vi "2_PTLF_Classification_Model_Converter.vi"() -> ()   [LabVIEW 2020]
uses:
  <vilib>/Ngene/DeepLTK FPGA Addon/Toolkit/NNF_Host/Low_Level/Network_Converter/Controls/Range_Calculation_Specs.ctl
  <vilib>/Ngene/Deep Learning Toolkit/Toolkit/NN_Network/Controls/NN_Device.ctl
  <vilib>/Ngene/Deep Learning Toolkit/Toolkit/Deep_Learning_Toolkit_by_Ngene.lvlib
  <vilib>/Ngene/DeepLTK FPGA Addon/Toolkit/DeepLTK_FPGA_Addon.lvlib
panel:
  in  "Dataset Path":path=path "D:/Ngene/GitHub/deepltk_fpga_examples/3_PTLF_Classification(PXI,sbRIO)/Dataset/Test"
  out "error out":errorcluster
  in  "Wights file":path=path "D:/Ngene/GitHub/deepltk_fpga_examples/3_PTLF_Classification(PXI,sbRIO)/Models/0_PTLF_Classification_Original/PTLF_Classifier_weights_24_11_21__13_37_15.bin"
  in  "Configuration file":path=path "D:/Ngene/GitHub/deepltk_fpga_examples/3_PTLF_Classification(PXI,sbRIO)/Models/0_PTLF_Classification_Original/PTLF_Classifier_net_cfg_24_11_21__13_37_15.cfg"
  out "Generated_Files":path[](array[path])
  in  "Dest":path=path "D:/Ngene/GitHub/deepltk_fpga_examples/3_PTLF_Classification(PXI,sbRIO)/Models/1_PTLF_Classification_Converted"
  # "Overview: This example demonstrates the preparation process of pretrained PTLF model to be deployed on FPGA.\nIt consists of the following stages:\n1. Network optimization by merging applicable layers together.\n2. Per layer weights and output statistics calculation for optimal quantization on FPGA.\n3. Saving converted model together with statistical information to be used during the deployment.\nRequirements:\n•DeepLTK - Deep Learning Toolkit for LabVIEW (https://www.ngene.co/deep-learning-toolkit-for-labview)\n•DeepLTK FPGA Addon(https://www.ngene.co/deepltk-accelerator-for-fpga)\n•Sample dataset for reliable output statistic calculation. \nInstructions: \n1.\tProvide the path to the configuration file of a pretrained model in the \"Configuration File\" control.\n2.\tProvide the path to the weights file of a pretrained model in the \"Weights File\" control. \n3.\tProvide the path to the MNIST dataset used during training in the \"Dataset Path\" control. \n4.\tProvide the destination directory where the results will be stored in the \"Dest\" control.\n5.\tRun the VI and wait until all processes are completed.\n\nThe resulting files (Scalers .cfg, Weights .bin, and Configuration .cfg) will be stored at paths displayed in \"Generated_Files\" indicator.\nThis files will be used during inference process.\nMore Examples: https://github.com/ngenehub/deepltk_fpga_examples"
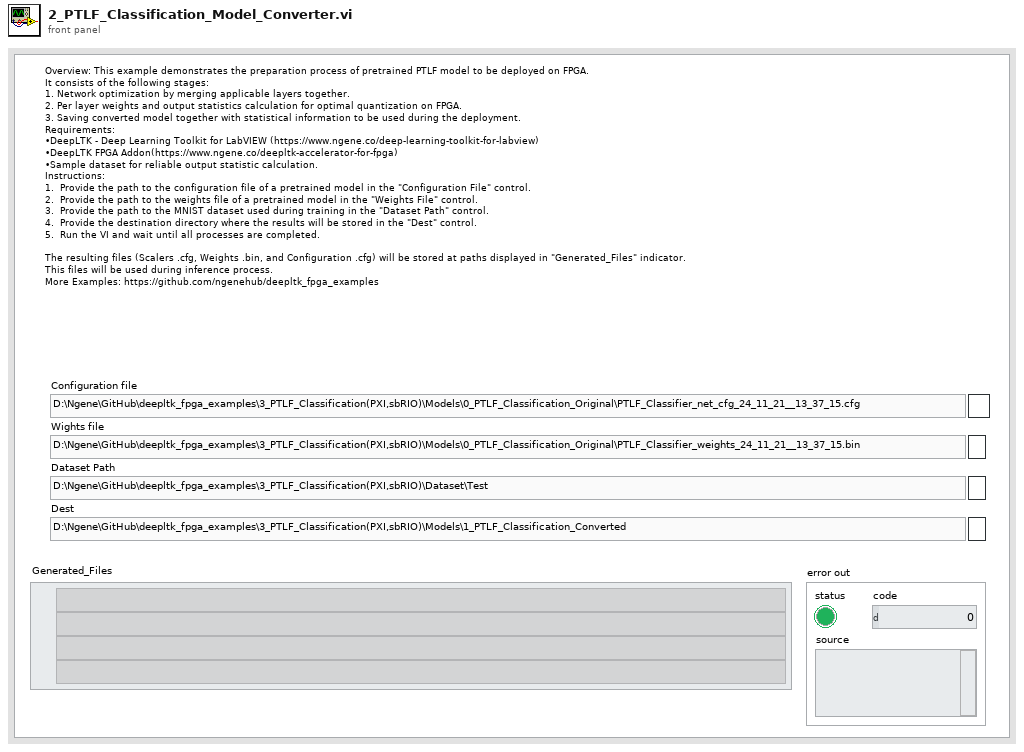
[diagram p1: front panel]
types:
  T1 = typedef "DeepLTK_FPGA_Addon.lvlib/Range_Calculation_Specs.ctl" = cluster{"# of Histogram Bins":i32, "Outputs Range Percentile(0.9999)":dbl, "Weights Range Percentile(0.9999)":dbl}
  T2 = typedef "Deep_Learning_Toolkit_by_Ngene.lvlib/NN_Device.ctl" = enum16{"CPU", "GPU"}
  T3 = typedef "Deep_Learning_Toolkit_by_Ngene.lvlib/NN_DataSets_All(In1D_Out1D).ctl" = cluster{"Train":T4, "Validation":T4, "Test":T4}
  T4 = typedef "Deep_Learning_Toolkit_by_Ngene.lvlib/NN_DataSet(In1D_Out1D).ctl" = cluster{"Inputs Ref.":variant, "Outputs Ref.":T5, "Dims_In":i32, "Dataset_Size":i32, "Dims_Out":i32, "Labels":string[], "File Paths":path[]}
  T5 = typedef "Deep_Learning_Toolkit_by_Ngene.lvlib/NN_Data_ref(2D_SGL).ctl" = refnum<data-value>
  T6 = typedef "Deep_Learning_Toolkit_by_Ngene.lvlib/NN_Config_Params.ctl" = cluster{"Name":string, "mBatch":i32, "NN_Train_Params":T7, "LR_Decay_Policy":T10, "Labels":string[], "Loss":T12}
  T7 = typedef "Deep_Learning_Toolkit_by_Ngene.lvlib/NN_Train_Params.ctl" = cluster{"Optimizer":T8, "Beta_1":sgl, "Beta_2":sgl, "Weight Decay(L1)":sgl, "Weight Decay(L2)":sgl, "Data_Sampling":T9}
  T8 = typedef "Deep_Learning_Toolkit_by_Ngene.lvlib/NN_Train_Optimizer.ctl" = enum16{"SGD", "Adam", "Adagrad", "Adadelta", "RMSProp", "Nesterov"}
  T9 = typedef "Deep_Learning_Toolkit_by_Ngene.lvlib/NN_Train_Data_Sampling.ctl" = enum16{"Random", "Sequential"}
  T10 = typedef "Deep_Learning_Toolkit_by_Ngene.lvlib/NN_LR_Policy_Cfg.ctl" = cluster{"Policy_Type":T11, "LR0":dbl, "k":sgl, "WarmUp_Policy":enum16{"Step", "Ramp"}, "WarmUp_Iter":i32, "WarmUp_Ratio":sgl}
  T11 = typedef "Deep_Learning_Toolkit_by_Ngene.lvlib/NN_LR_Policy_Type.ctl" = enum16{"Manual", "Step", "Exp", "1/t"}
  T12 = typedef "Deep_Learning_Toolkit_by_Ngene.lvlib/NN_Loss_Config_Params.ctl" = cluster{"Loss_Type":T13, "Loss_Conf_Params":variant}
  T13 = typedef "Deep_Learning_Toolkit_by_Ngene.lvlib/NN_Loss_Type.ctl" = enum16{"None", "MSE", "CrossEntropy", "YOLO_v2", "YOLO_v4"}
  T14 = typedef "Deep_Learning_Toolkit_by_Ngene.lvlib/NN_Layer_Config_Params.ctl" = cluster{"Layer_Type":T15, "Layer_Conf_Params":variant, "Input Layers":string[]}
  T15 = typedef "Deep_Learning_Toolkit_by_Ngene.lvlib/NN_Layer_Type.ctl" = enum16{"Input1D", "Input3D", "Conv1D", "Conv2D", "Conv2D_Adv", "MaxPool", "AvgPool", "UpSample", "DropOut3D", "ShortCut", "Concat", "SoftMax3D", "FC", "DropOut", "Softmax", "Flatten", "YOLO_v2", "YOLO_v4", "Activation", "BatchNormalization", "Unsupported"}
  T16 = typedef "Deep_Learning_Toolkit_by_Ngene.lvlib/NN.ctl" = cluster{"Name":string, "No of Layers":i32, "mBatch":i32, "Layers":T17[], "Dimty":T18, "Dims_In":T19, "Dims_Out":T19, "Working_Dir":path, "Train?":bool, "Train_Params":T7, "LR_Update_Policy":T10, "Session Data":T20, "Ground_truth":T21, "NNg_hdls":T22, "NN_Device":T2, "GPU Id":i32, "Labels":string[], "Receptive Field":T23[], "Loss_Type":T13, "Loss_Cfg_Prms":variant, "NNG_WS":T24}
  T17 = typedef "Deep_Learning_Toolkit_by_Ngene.lvlib/NN_Layer_ref.ctl" = refnum<data-value>
  T18 = typedef "Deep_Learning_Toolkit_by_Ngene.lvlib/NN_In_Out_Dim-ty.ctl" = enum8{"In1D_Out1D", "In3D_Out1D", "In3D_Out3D", "In3D_OutBBox"}
  T19 = typedef "Deep_Learning_Toolkit_by_Ngene.lvlib/NN_Dims(C,H,W).ctl" = cluster{"C":i32, "H":i32, "W":i32}
  T20 = typedef "Deep_Learning_Toolkit_by_Ngene.lvlib/NN_Train_Session_Data.ctl" = cluster{"Epochs":sgl, "Tot_Iter":i32, "LR":sgl, "LR_iter":i32}
  T21 = typedef "Deep_Learning_Toolkit_by_Ngene.lvlib/NN_Ground_truth.ctl" = cluster{"Y":variant}
  T22 = typedef "Deep_Learning_Toolkit_by_Ngene.lvlib/nng_cuda_handles.ctl" = cluster{"cudnn":u64, "cublas":u64, "stream":u64, "curand":u64}
  T23 = typedef "Deep_Learning_Toolkit_by_Ngene.lvlib/NN_Dims(V,H).ctl" = cluster{"V":i32, "H":i32}
  T24 = typedef "Deep_Learning_Toolkit_by_Ngene.lvlib/NNG_WS.ctl" = cluster{"NNG_WS_Mem":T25, "Max_WS_Size":i64}
  T25 = typedef "Deep_Learning_Toolkit_by_Ngene.lvlib/NNg_WS_Mem_DVR.ctl" = refnum<data-value>
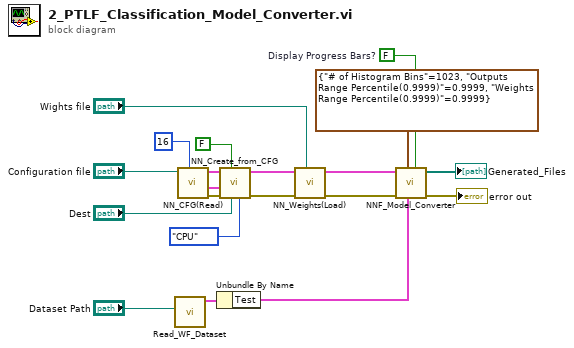
[diagram p0: block diagram]
diagram:
  w1 = FALSE  # Display Progress Bars?
  n1 = call "Read_WF_Dataset.vi"("Test dataset path"="Dataset Path") -> ("NN_Dataset"=w9:T3)  [unwired: 10 in]
  n2 = call <vilib>:"NN_CFG(Read).vi"("mBatch"=16, "CFG file path"="Configuration file") -> ("error out"=w17:errorcluster, "Net_Cfg"=w20:T6, "Layer_Cfg"=w16:T14[])  [unwired: 7 in]
  n3 = Unbundle By Name(w9) -> ("Test"=w8:T4)
  n4 = call <vilib>:"NN_Create_from_CFG.vi"("NN_Device"=NN_Device."CPU", "Working Dir"="Dest", "Train? (false)"=FALSE, "error in (no error)"=w17, "Net_Cfg"=w20, "Layer_Cfg"=w16) -> ("error out"=w18:errorcluster, "NN out"=w19:T16)  [unwired: 4 in]
  n5 = call <vilib>:"NN_Weights(Load).vi"("Weight File Path"="Wights file", "error in (no error)"=w18, "NN in"=w19) -> ("error out"=w12:errorcluster, "NN out"=w13:T16)  [unwired: 7 in]
  n6 = call <vilib>:"NNF_Model_Converter.vi"("Display Progress Bars?"=w1, "DataSet"=w8, "Range_Calculation_Specs"=T1 {"# of Histogram Bins"=1023, "Outputs Range Percentile(0.9999)"=0.9999, "Weights Range Percentile(0.9999)"=0.9999}, "error in (no error)"=w12, "NN in"=w13) -> ("error out"=→"error out":errorcluster, "Generated_Files"=→"Generated_Files":path[])  [unwired: 3 in, 2 out]
